vi "LowPassFilter.vi"(8 "error in (no error)":errorcluster, 9 "Àcquiring Configurations":T1={"Accel-ai0"=FALSE, "Maximum Input"=0.0, "Minimum Input"=0.0, "HW Sample Rate"=0.0, "SW Sample Rate"=0.0, "Number of Samples"=0, "Accel-ai1"=FALSE, "DAQmx Task"="", "Low Pass Filter"={"Upper Cutoff"=350.0, "Lower Cutoff"=5.0, "Order"=3}} {"Low Pass Filter"."Order" min=0 max=10 step=1}, 11 "InputData":waveform(dbl)[](array[waveform])) -> (0 "error out":errorcluster, 3 "OutputData":waveform(dbl)[](array[waveform]))   [LabVIEW 2022 SP3]
uses:
  FiniteMeasurement-DAQmx/controls/Hardware Configuration.ctl
  AcquisitionFilter.ctl
  <vilib>/Analysis/3filter.llb/Filter Passband Type.ctl
  <vilib>/Analysis/3filter.llb/Butterworth Filter (DBL).vi
  <vilib>/Analysis/NI_AALBase.lvlib
  Acquisition/Acquisition.lvlib
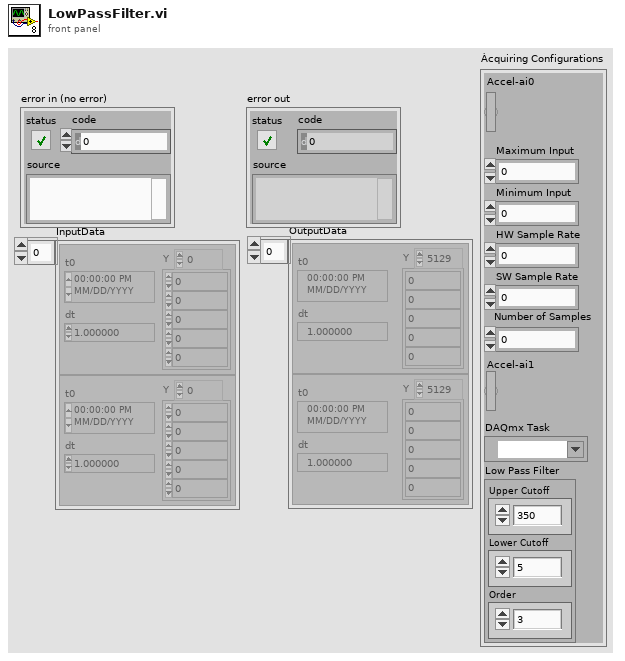
[diagram p1: front panel]
types:
  T1 = typedef "Acquisition.lvlib/Hardware Configuration.ctl" = cluster{"Accel-ai0":bool, "Maximum Input":dbl, "Minimum Input":dbl, "HW Sample Rate":dbl, "SW Sample Rate":dbl, "Number of Samples":i32, "Accel-ai1":bool, "DAQmx Task":refnum<k21>, "Low Pass Filter":T2}
  T2 = typedef "Acquisition.lvlib/AcquisitionFilter.ctl" = cluster{"Upper Cutoff":dbl, "Lower Cutoff":dbl, "Order":i32}
  T3 = typedef "NI_AALBase.lvlib/Filter Passband Type.ctl" = enum32{"Lowpass", "Highpass", "Bandpass", "Bandstop"}
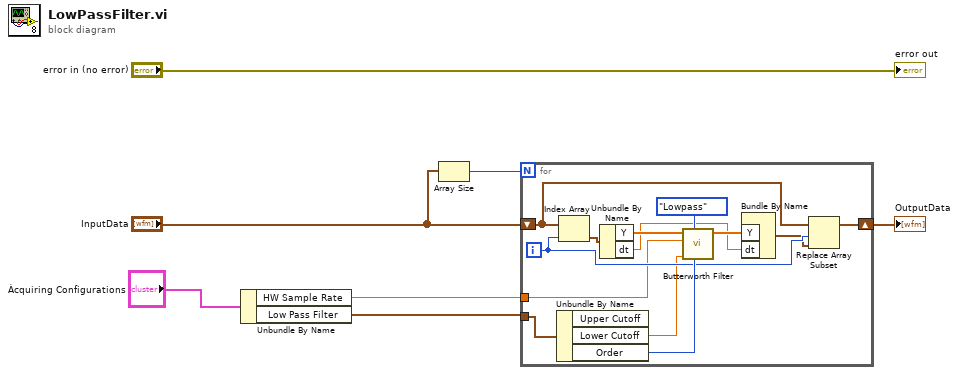
[diagram p0: block diagram]
diagram:
  n1 = Unbundle By Name("Àcquiring Configurations") -> ("HW Sample Rate"=w2:dbl, "Low Pass Filter"=w1:T2)
  n2 = Array Size(array="InputData") -> (size(s)=w7:i32)
  n3 = for {
    N: w7 -> [_]
    tunnel: w1 -> [w15]
    shift-right: [w20] -> w3
    shift-left: "InputData" -> [w11]
    tunnel: w2 -> [w9]
    i -> [w13]
    n4 = Unbundle By Name(w15) -> ("Lower Cutoff"=w8:dbl, "Order"=w14:i32)  [unwired: 1 out]
    n5 = Index Array(array=w11, index=w13) -> (element=w17:waveform(dbl))
    n6 = Unbundle By Name(w17) -> ("Y"=w19:dbl[], "dt"=w10:dbl)
    n7 = call-poly <vilib>:"Butterworth Filter.vi"("order"=w14, "filter type"=Filter_Passband_Type."Lowpass", "low cutoff freq: fl"=w8, "sampling freq: fs"=w9, "X"=w19) -> ("Filtered X"=w16:dbl[])  [unwired: 3 in, 1 out]
    n8 = Bundle By Name("Y"=w16, "dt"=w10) -> (w12:waveform(dbl))  [unwired: 1 in]
    n9 = Replace Array Subset(array=w11, new element=w12, index=w13) -> (w20:waveform(dbl)[])
  }
  "OutputData" <- w3
  "error out" <- "error in (no error)"
